vi "BRig_dataExp_Audio_pattern_L.vi"() -> (2 "output_Audio_sp__L":i32)   [LabVIEW 2014]
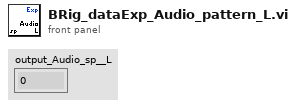
[diagram p1: front panel]
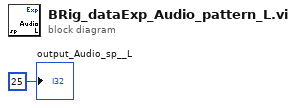
[diagram p0: block diagram]
diagram:
  "output_Audio_sp__L" <- 25 ("output_iBlock")
